vi "create.vi"(9 "Description":string, 10 "Name":string) -> (3 "dataset":refnum<class "dataset.lvclass">)   [LabVIEW 2020, in "datasources.lvlib" / "dataset.lvclass"]
uses:
  dataset.lvclass
  dataset.lvclass/dataset.ctl
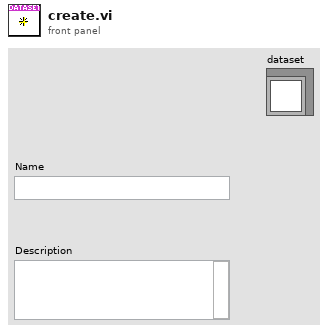
[diagram p1: front panel]
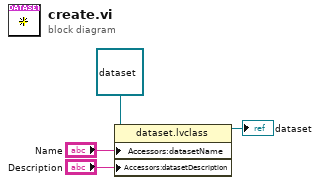
[diagram p0: block diagram]
diagram:
  n1 = property class="dataset.lvclass"(reference=refnum<class "dataset.lvclass"> refnum ("datasources.lvlib:dataset.lvclass"), "Accessors:datasetName"="Name", "Accessors:datasetDescription"="Description") -> (reference out=→"dataset":refnum<class "dataset.lvclass">)  [unwired: 1 in, 1 out]
